vi "PositionVideo.vi"() -> ()   [LabVIEW 2012]
uses:
  <userlib>/_OpenG.lib/array/array.llb/Empty 1D Array (DBL)__ogtk.vi
panel:
  in  "LabVIEW file?":bool
  in  "Mode?":enum16{"Overlay", "Extend"}(ring)
  in  "Interframe time (s)":dbl
  in  "Image file pattern":string="*tif*"
  out "error out":errorcluster
  in  "error in (no error)":errorcluster
  in  "Positions file":path
  in  "Output images folder":path
  in  "Input images folder":path
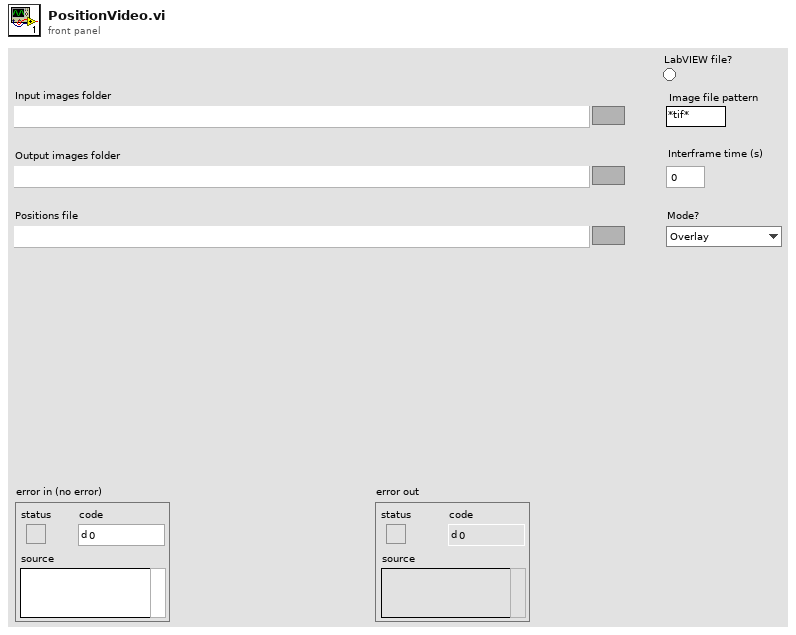
[diagram p1: front panel]
types:
  T1 = typedef "IMAQ Image.ctl" = refnum<image>
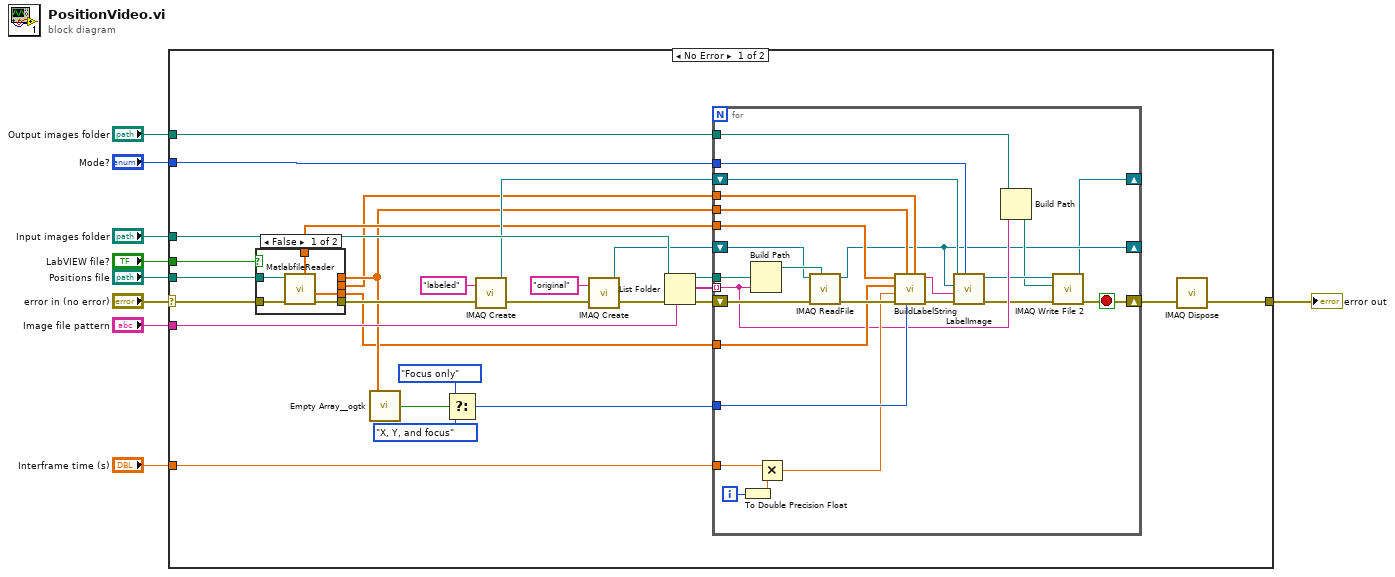
[diagram p0: block diagram]
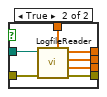
[diagram p2: hidden frame]
diagram:
  n1 = case shown="No Error" "error in (no error)" {
    selector: "error in (no error)" -> [w32 w76]
    tunnel: [w11 w76] -> w8
    tunnel: "Input images folder" -> [w37 _]
    tunnel: "Image file pattern" -> [w36 _]
    tunnel: "Positions file" -> [w31 _]
    tunnel: "Interframe time (s)" -> [w15 _]
    tunnel: "Mode?" -> [w14 _]
    tunnel: "Output images folder" -> [w13 _]
    tunnel: "LabVIEW file?" -> [w10 _]
    frame No Error {
      n2 = case shown="False" w10 {
        tunnel: w32 -> [w42 w49]
        tunnel: w31 -> [w41 w48]
        tunnel: [w40 w47] -> w29
        tunnel: [w38 w46] -> w19
        tunnel: [_ w45] -> w18
        tunnel: [_ w44] -> w17
        tunnel: [w39 w43] -> w16
        frame False {
          n3 = call "MatlabfileReader.vi"("error in (no error)"=w42, "Positions file"=w41) -> ("error out"=w40:errorcluster, "Focus"=w39:dbl[], "Time"=w38:dbl[])  [unwired: 5 in, 2 out]
        }
        frame True {
          n4 = call "LogfileReader.vi"("error in (no error)"=w49, "Positions file"=w48) -> ("error out"=w47:errorcluster, "Focus"=w43:dbl[], "Y"=w44:dbl[], "X"=w45:dbl[], "Time"=w46:dbl[])  [unwired: 5 in]
        }
      }
      n5 = call-poly <userlib>:"Empty Array__ogtk.vi"("Array"=w18) -> ("Empty Array?"=w22:bool)  [unwired: 8 in]
      n6 = Select(t=enum16{"Focus only", "X, Y, and focus"}."Focus only" ("Axes"), s=w22, f=enum16{"Focus only", "X, Y, and focus"}."X, Y, and focus" ("Axes")) -> (s? t:f=w20:enum16{"Focus only", "X, Y, and focus"})
      n7 = call "IMAQ Create"("Image Name"="labeled", "error in (no error)"=w29) -> ("New Image"=w25:T1, "error out"=w30:errorcluster)  [unwired: 3 in]
      n8 = call "IMAQ Create"("Image Name"="original", "error in (no error)"=w30) -> ("New Image"=w24:T1, "error out"=w28:errorcluster)  [unwired: 3 in]
      n9 = List Folder(path=w37, pattern=w36, error in=w28) -> (path out=w34:path, filenames=w33:string[], error out=w35:errorcluster)  [unwired: 1 in, 1 out]
      n10 = for {
        shift-right: [w50] -> w12
        shift-left: w35 -> [w74]
        tunnel: w34 -> [w75]
        tunnel: w33 -> [w56] mode=indexing
        tunnel: w20 -> [w71]
        tunnel: w19 -> [w68]
        tunnel: w18 -> [w67]
        tunnel: w17 -> [w66]
        tunnel: w16 -> [w65]
        tunnel: w15 -> [w62]
        tunnel: w14 -> [w58]
        tunnel: w13 -> [w57]
        shift-right: [w51] -> _
        shift-left: w25 -> [w59]
        shift-right: [w52] -> _
        shift-left: w24 -> [w72]
        i -> [w64]
        stop <- w50 stop-if-true
        n11 = To Double Precision Float(number=w64) -> (double precision float=w63:dbl)
        n12 = Build Path(base path=w75, name or relative path=w56) -> (appended path=w73:path)
        n13 = Multiply(x=w62, y=w63) -> (x*y=w61:dbl)
        n14 = call "IMAQ ReadFile"("File Path"=w73, "error in (no error)"=w74, "Image"=w72) -> ("error out"=w70:errorcluster, "Image Out"=w52:T1)  [unwired: 4 in, 3 out]
        n15 = call "BuildLabelString.vi"("Y"=w66, "Axes"=w71, "X"=w67, "error in (no error)"=w70, "Image time"=w61, "Focus"=w65, "Time array"=w68) -> ("error out"=w69:errorcluster, "Label string"=w60:string)  [unwired: 3 in]
        n16 = call "LabelImage.vi"("Mode?"=w58, "error in (no error)"=w69, "Label"=w60, "Original image in"=w52, "Labeled image in"=w59) -> ("error out"=w55:errorcluster, "Labeled image out"=w54:T1)  [unwired: 4 in, 1 out]
        n17 = Build Path(base path=w57, name or relative path=w56) -> (appended path=w53:path)
        n18 = call-poly "IMAQ Write File 2"("error in (no error)"=w55, "File Path"=w53, "Image"=w54) -> ("error out"=w50:errorcluster, "Image Out (duplicate)"=w51:T1)  [unwired: 7 in]
      }
      n19 = call "IMAQ Dispose"("error in (no error)"=w12) -> ("error out"=w11:errorcluster)  [unwired: 5 in]
    }
    frame Error {
    }
  }
  "error out" <- w8
